vi "config.vi"(7 "FUN":enum16{"R", "W"}(ring), 8 "error in (no error)":errorcluster caption="错误输入（无错误）", 11 "配置输入":T1={"AD通道"=enum."AD2", "K"=0.000305213, "b"=-0.5, "修正系数"=1.0, "数据保存间隔"=60}) -> (0 "error out":errorcluster caption="错误输出", 3 "配置输出":T1={"AD通道"=enum."AD2", "K"=0.000305213, "b"=-0.5, "修正系数"=1.0, "数据保存间隔"=60})   [LabVIEW 2016, in "余氯.lvlib"]
uses:
  <vilib>/Utility/config.llb/NI_LVConfig.lvlib
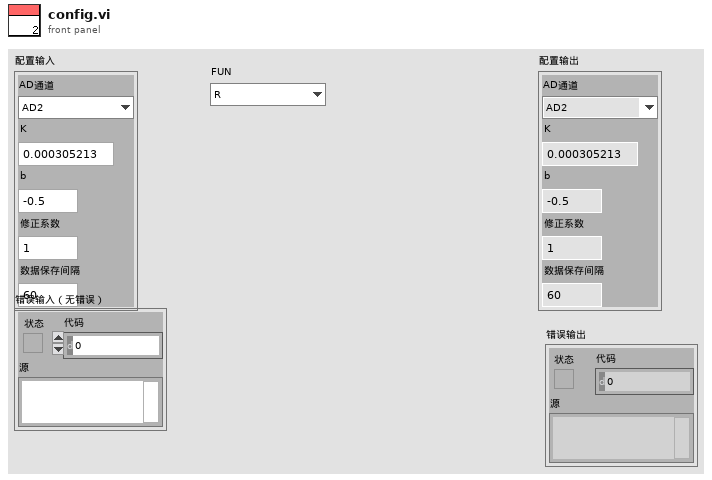
[diagram p1: front panel]
types:
  T1 = cluster{"AD通道":enum16{"AD0", "AD1", "AD2", "AD3", "AD4", "AD5"}, "K":dbl, "b":dbl, "修正系数":dbl, "数据保存间隔":i32}
  T2 = typedef "NI_LVConfig.lvlib/Config Data RefNum.ctl" = refnum<k1>
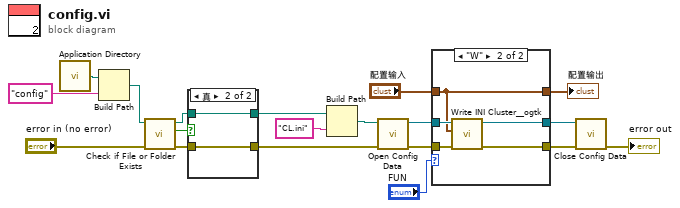
[diagram p0: block diagram]
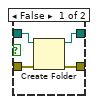
[diagram p2: hidden frame]
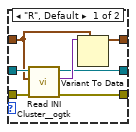
[diagram p3: hidden frame]
diagram:
  n1 = call <vilib>:"Application Directory.vi"() -> ("Application Directory"=w12:path)
  n2 = Build Path(base path=w12, name or relative path="config" ("名称或相对路径")) -> (appended path=w10:path)
  n3 = call <vilib>:"Check if File or Folder Exists.vi"("error in (no error)"="error in (no error)", "path"=w10) -> ("error out"=w3:errorcluster, "file or folder exists?"=w9:bool, "dup path"=w8:path)  [unwired: 7 in]
  n4 = case shown="真" w9 {
    tunnel: w8 -> [w23 w25]
    tunnel: [w22 w25] -> w7
    tunnel: [w21 w24] -> w4
    tunnel: w3 -> [w20 w24]
    frame False {
      n5 = Create Folder(path (use dialog)=w23, error in=w20) -> (created path=w22:path, error out=w21:errorcluster)  [unwired: 1 in, 1 out]
    }
    frame True {
    }
  }
  n6 = Build Path(base path=w7, name or relative path="CL.ini" ("名称或相对路径")) -> (appended path=w6:path)
  n7 = call <vilib>:"Open Config Data.vi"("error in (no error)"=w4, "configuration file path"=w6) -> ("error out"=w17:errorcluster, "refnum"=w19:T2)  [unwired: 7 in, 1 out]
  n8 = case shown="\"W\"" "FUN" {
    tunnel: w19 -> [w32 w37]
    tunnel: "配置输入" -> [w29 w33]
    tunnel: w17 -> [w31 w36]
    tunnel: [w27 w35] -> w14
    tunnel: [w26 w34] -> w13
    tunnel: [w28 w33] -> w15
    frame "R", Default {
      n9 = call <userlib>:"Read INI Cluster__ogtk.vi"("error in (no error)"=w31, "INI Fomatted Cluster Type"=w29, "refnum"=w32) -> ("error out"=w26:errorcluster, "INI Fomatted Cluster"=w30:variant, "dup refnum"=w27:T2)  [unwired: 4 in, 2 out]
      n10 = Variant To Data(type=w29, Variant=w30) -> (data=w28:T1)  [unwired: 1 in, 1 out]
    }
    frame "W" {
      n11 = call <userlib>:"Write INI Cluster__ogtk.vi"("error in (no error)"=w36, "INI Fomatted Cluster"=w33, "refnum"=w37) -> ("error out"=w34:errorcluster, "dup refnum"=w35:T2)  [unwired: 7 in]
    }
  }
  "配置输出" <- w15
  n12 = call <vilib>:"Close Config Data.vi"("error in (no error)"=w13, "refnum"=w14) -> ("error out"=→"error out":errorcluster)  [unwired: 8 in, 1 out]
